vi "Persist Test.vi"() -> ()   [LabVIEW 2020]
uses:
  <vilib>/gpm_packages/@cs/data-type-serializer/source/I32/I32.lvclass/I32.ctl
  <vilib>/gpm_packages/@cs/data-type-serializer/source/Boolean/Boolean.lvclass/Boolean.ctl
  <vilib>/gpm_packages/@cs/persistence/source/XML/XML.lvclass
  <vilib>/gpm_packages/@cs/persistence/source/CAML/CAML.lvclass
  C:/Program Files/National Instruments/LabVIEW 2020/vi.lib/gpm_packages/@cs/persistence/source/IPersist/IPersist.lvclass
  <vilib>/gpm_packages/@cs/linked-list/Source/Linked List/Linked List/Linked List.lvclass
  C:/Program Files/National Instruments/LabVIEW 2020/vi.lib/gpm_packages/@cs/linked-list/Source/Linked List/ILinkedList/ILinked List.lvclass
  <vilib>/gpm_packages/@cs/data-type-serializer/source/I32/I32.lvclass
  C:/Program Files/National Instruments/LabVIEW 2020/vi.lib/gpm_packages/@cs/data-type-serializer/source/Data Type/Data Type.lvclass
  e6fe5fcf-7207-4b44-b52c-de58ab45d0de.vi
  c032021d-faa0-478d-8805-bec44217c56e.vi
  3dcc5633-58d3-425a-bfbd-c9ba4060836c.vi
  <vilib>/gpm_packages/@cs/data-type-serializer/source/Boolean/Boolean.lvclass
  <vilib>/gpm_packages/@cs/linked-list/Source/Linked List/ILinkedList/ILinked List.lvclass
  <vilib>/gpm_packages/@cs/linked-list/Source/Linked List/Linked List Ref/Linked List Ref.lvclass
panel:
  out "Found?":bool
  out "I32 out":i32
  in  "Tree 2":string(tree)
  in  "File Name":string
  in  "Folder":path
  in  "Tree":string(tree)
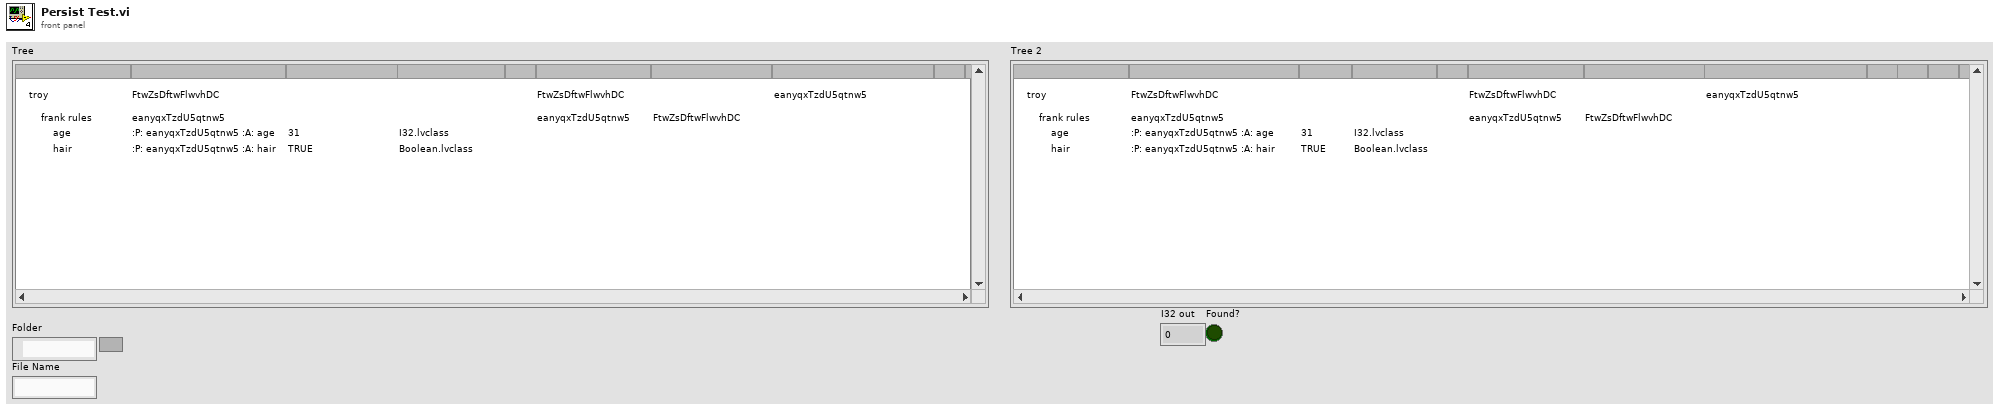
[diagram p1: front panel]
types:
  T1 = cluster{"Left Cell String":string, "Child Text":string[], "Child Tag":string, "Item Indent":i32, "Child Only?":bool, "Glyph Index":i32}[]
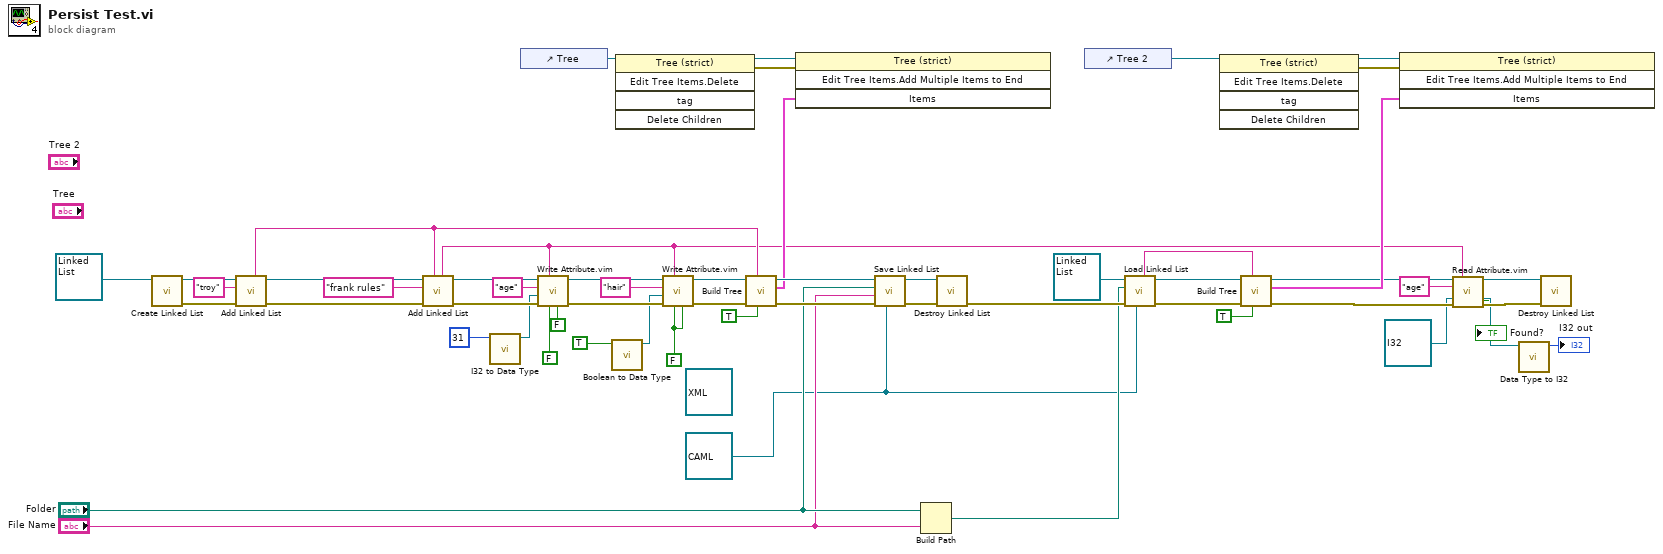
[diagram p0: block diagram]
diagram:
  w15 = FALSE ("Pointer?")
  w1 = refnum<class "CAML.lvclass"> refnum ("CAML.lvlib:CAML.lvclass")
  (unwired) refnum<class "XML.lvclass"> refnum ("XML.lvlib:XML.lvclass")
  n1 = call <vilib>:"Create Linked List.vi"("Linked List"=refnum<class "Linked List.lvclass"> refnum ("Dictionary.lvlib:Dictionary.lvclass")) -> ("error out"=w46:errorcluster, "Linked List Ref"=w48:refnum<data-value>)  [unwired: 9 in]
  n2 = call <vilib>:"Add Linked List.vi"("error in (no error)"=w46, "Name"="troy" ("Dictionary Name"), "Linked List Ref"=w48) -> ("error out"=w45:errorcluster, "Linked List Ref out"=w47:refnum<data-value>, "Linked List ID out"=w37:string)  [unwired: 5 in, 1 out]
  n3 = call <vilib>:"Add Linked List.vi"("Parent ID"=w37, "error in (no error)"=w45, "Name"="frank rules", "Linked List Ref"=w47) -> ("error out"=w53:errorcluster, "Linked List Ref out"=w54:refnum<data-value>, "Linked List ID out"=w2:string)  [unwired: 4 in, 1 out]
  n4 = call <vilib>:"I32 to Data Type.vi"("I32"=31) -> ("Boolean out"=w42:refnum<class "I32.lvclass">)  [unwired: 9 in, 1 out]
  n5 = control-ref of="Tree"() -> (w31:refnum<vi>)
  n6 = call "Write Attribute.vim"("Private?"=FALSE, "Pointer?"=FALSE, "Linked List ID"=w2, "error in (no error)"=w53, "Attribute"=w42, "Attribute Name"="age", "Linked List Ref"=w54) -> ("error out"=w50:errorcluster, "Linked List Ref out"=w51:refnum<data-value>)  [unwired: 1 in, 2 out]
  n7 = call <vilib>:"Boolean to Data Type.vi"("Boolean"=TRUE) -> ("Boolean out"=w40:refnum<class "Boolean.lvclass">)  [unwired: 9 in, 1 out]
  n8 = invoke on="Invoke Node" class="Tree (strict)" method="Edit Tree Items.Delete"(reference=w31) -> (reference out=w29:refnum<vi>, error out=w32:errorcluster)  [unwired: 4 in, 3 out]
  n9 = call "Write Attribute.vim"("Private?"=w15, "Pointer?"=w15, "Linked List ID"=w2, "error in (no error)"=w50, "Attribute"=w40, "Attribute Name"="hair", "Linked List Ref"=w51) -> ("error out"=w38:errorcluster, "Linked List Ref out"=w39:refnum<data-value>)  [unwired: 1 in, 2 out]
  n10 = call <vilib>:"Build Tree.vi"("Show IDs"=TRUE, "Linked List ID"=w37, "error in (no error)"=w38, "Linked List Ref"=w39) -> ("error out"=w34:errorcluster, "Tree Data"=w30:T1, "Linked List Ref out"=w36:refnum<data-value>)  [unwired: 5 in]
  n11 = invoke on="Invoke Node" class="Tree (strict)" method="Edit Tree Items.Add Multiple Items to End"(reference=w29, error in=w32, "Items"=w30) -> ()  [unwired: 1 in, 4 out]
  n12 = call <vilib>:"Save Linked List.vi"("Persistence"=w1, "error in (no error)"=w34, "File Name"="File Name", "Folder"="Folder", "Linked List Ref"=w36) -> ("error out"=w33:errorcluster, "Linked List Ref out"=w35:refnum<data-value>)  [unwired: 5 in]
  n13 = Build Path(base path="Folder", name or relative path="File Name") -> (appended path=w21:path)
  n14 = call <vilib>:"Destroy Linked List.vi"("error in (no error)"=w33, "Linked List Ref"=w35) -> ("error out"=w25:errorcluster)  [unwired: 9 in]
  n15 = control-ref of="Tree 2"() -> (w18:refnum<vi>)
  n16 = call <vilib>:"Load Linked List.vi"("Persistence"=w1, "error in (no error)"=w25, "File Path"=w21, "Linked List"=refnum<class "Linked List.lvclass"> refnum ("Dictionary.lvlib:Dictionary.lvclass")) -> ("error out"=w26:errorcluster, "Linked List Ref out"=w27:refnum<data-value>, "Linked List ID out"=w8:string)  [unwired: 5 in]
  n17 = invoke on="Invoke Node" class="Tree (strict)" method="Edit Tree Items.Delete"(reference=w18) -> (reference out=w20:refnum<vi>, error out=w19:errorcluster)  [unwired: 4 in, 3 out]
  n18 = call <vilib>:"Build Tree.vi"("Show IDs"=TRUE, "Linked List ID"=w8, "error in (no error)"=w26, "Linked List Ref"=w27) -> ("error out"=w10:errorcluster, "Tree Data"=w17:T1, "Linked List Ref out"=w12:refnum<data-value>)  [unwired: 5 in]
  n19 = invoke on="Invoke Node" class="Tree (strict)" method="Edit Tree Items.Add Multiple Items to End"(reference=w20, error in=w19, "Items"=w17) -> ()  [unwired: 1 in, 4 out]
  n20 = call "Read Attribute.vim"("Linked List Ref"=w12, "Linked List ID"=w2, "Attribute Name"="age", "Type"=refnum<class "I32.lvclass"> refnum ("I32.lvclass"), "error in (no error)"=w10) -> ("Linked List Ref out"=w11:refnum<data-value>, "Attribute"=w5:refnum<class "I32.lvclass">, "Found?"=→"Found?":bool, "error out"=w9:errorcluster)  [unwired: 5 in, 2 out]
  n21 = call <vilib>:"Data Type to I32.vi"("Data Type"=w5) -> ("I32 out"=→"I32 out":i32)  [unwired: 9 in, 1 out]
  n22 = call <vilib>:"Destroy Linked List.vi"("error in (no error)"=w9, "Linked List Ref"=w11) -> ()  [unwired: 9 in, 1 out]
